vi "get_sjbumen_juese.vi"(7 "juese":string, 8 "lc_num":string, 9 "data_name":string) -> (0 "didian":string, 1 "zc_luodi_num":string, 2 "gonghao":string, 3 "sjbumen":string, 4 "error":errorcluster caption="error out 4", 5 "error":errorcluster caption="error out 4")   [LabVIEW 2017, in "Lib_code.lvlib"]
uses:
  Lib_code.lvlib
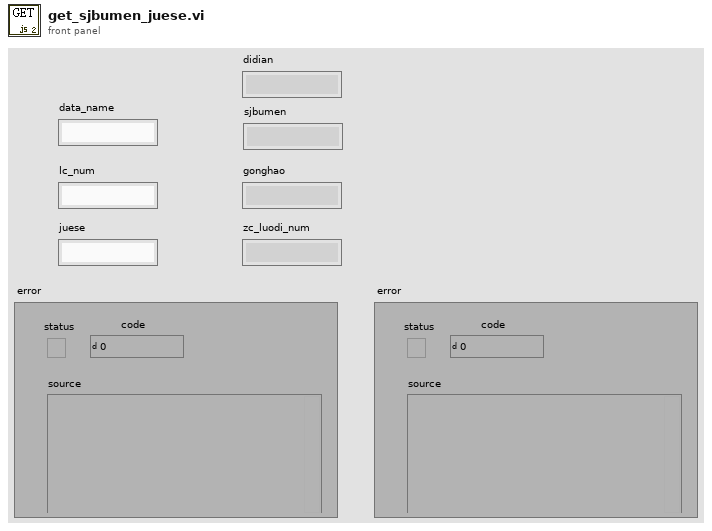
[diagram p1: front panel]
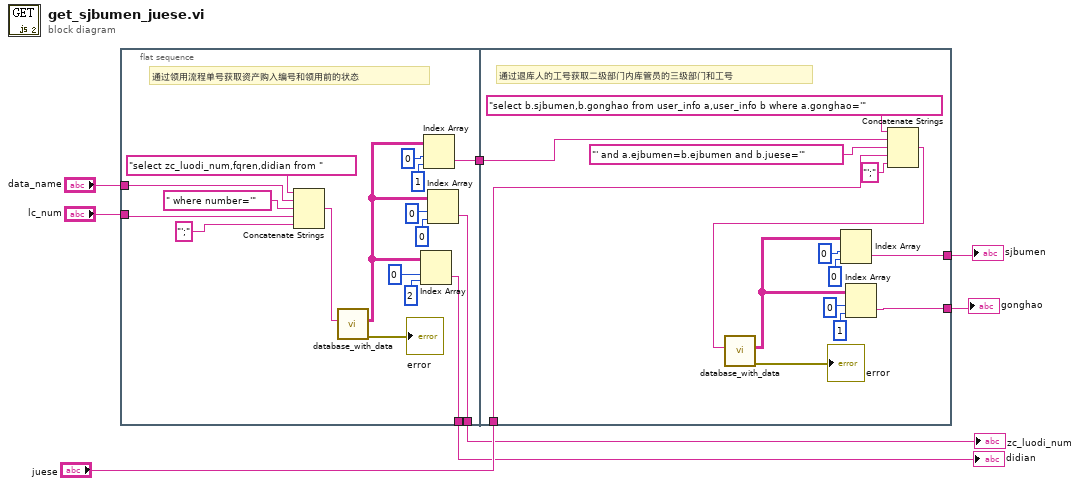
[diagram p0: block diagram]
diagram:
  n1 = flat-sequence {
    tunnel: "lc_num" -> [w23]
    tunnel: [w18] -> w8
    tunnel: "data_name" -> [w17]
    tunnel: [w10] -> w2
    tunnel: [w9] -> w1
    tunnel: w8 -> [w37]
    tunnel: [w32] -> w6
    tunnel: [w31] -> w5
    tunnel: "juese" -> [w30]
    frame #0 {
      # "通过领用流程单号获取资产购入编号和领用前的状态"
      n2 = Concatenate Strings("select zc_luodi_num,fqren,didian from " ("Command Text"), w17, " where number='" ("Command Text"), w23, "';" ("字符串")) -> (w15:string)
      n3 = call "database_with_data.vi"("input"=w15) -> ("error"=→"error":errorcluster, "Data"=w11:string[][])  [unwired: 9 in]
      n4 = Index Array(array=w11, index (row)=0 ("索引 (行)"), index (col)=2 ("禁用的索引 (列)")) -> (element=w10:string)
      n5 = Index Array(array=w11, index (row)=0 ("索引 (行)"), index (col)=1 ("禁用的索引 (列)")) -> (element=w18:string)
      n6 = Index Array(array=w11, index (row)=0 ("索引 (行)"), index (col)=0 ("禁用的索引 (列)")) -> (element=w9:string)
    }
    frame #1 {
      # "通过退库人的工号获取二级部门内库管员的三级部门和工号"
      n7 = Concatenate Strings("select b.sjbumen,b.gonghao from user_info a,user_info b where a.gonghao='" ("Command Text"), w37, "' and a.ejbumen=b.ejbumen and b.juese='" ("字符串"), w30, "';" ("字符串")) -> (w28:string)
      n8 = call "database_with_data.vi"("input"=w28) -> ("error"=→"error":errorcluster, "Data"=w27:string[][])  [unwired: 9 in]
      n9 = Index Array(array=w27, index (row)=0 ("索引 (行)"), index (col)=0 ("禁用的索引 (列)")) -> (element=w32:string)
      n10 = Index Array(array=w27, index (row)=0 ("索引 (行)"), index (col)=1 ("禁用的索引 (列)")) -> (element=w31:string)
    }
  }
  "gonghao" <- w5
  "sjbumen" <- w6
  "zc_luodi_num" <- w1
  "didian" <- w2
